vi "TEX_SIZE.vi"() -> (0 "TEX_SIZE":u32=4096)   [LabVIEW 2020]
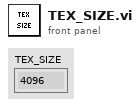
[diagram p1: front panel]
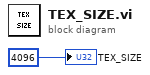
[diagram p0: block diagram]
diagram:
  "TEX_SIZE" <- u32 4096
